vi "acoustic moderm processing.vi"(8 "error in (no error)":errorcluster, 9 "WRITE BUTTON":bool, 11 "Cluster":T1) -> (0 "error in (no error) 2":errorcluster, 1 "Modem Ready Status":bool, 2 "Data Tx/Rx":string, 3 "Data out":string)   [LabVIEW 2021]
panel:
  out "concatenated string":string
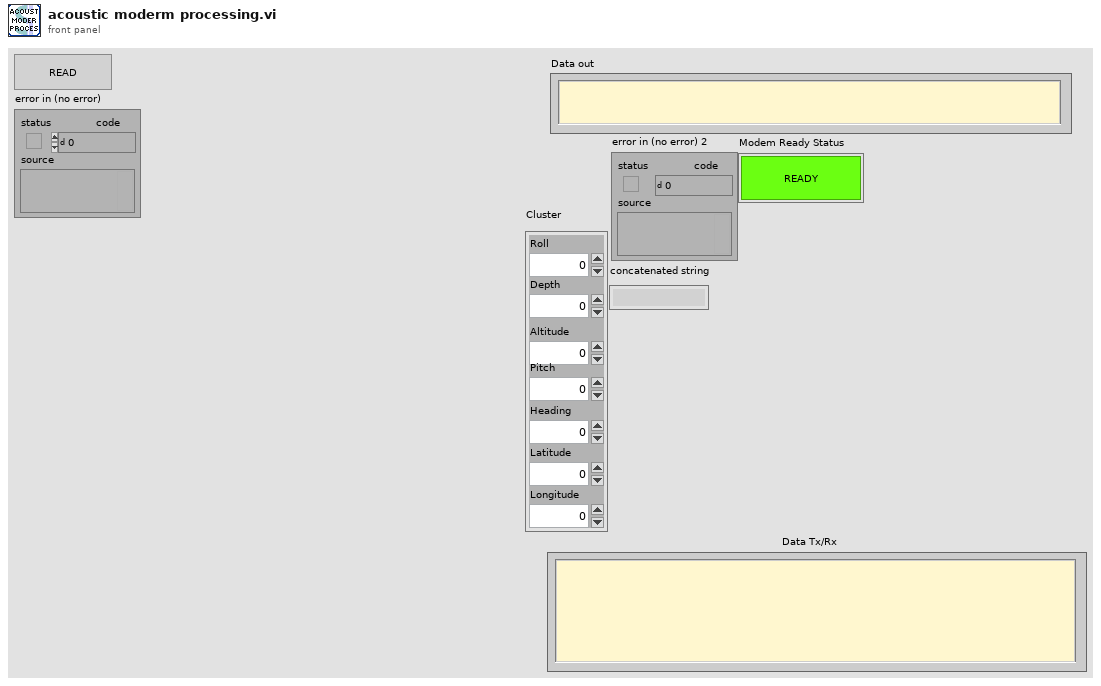
[diagram p1: front panel]
types:
  T1 = cluster{"Roll":sgl, "Depth":sgl, "Altitude":sgl, "Pitch":sgl, "Heading":sgl, "Latitude":sgl, "Longitude":sgl}
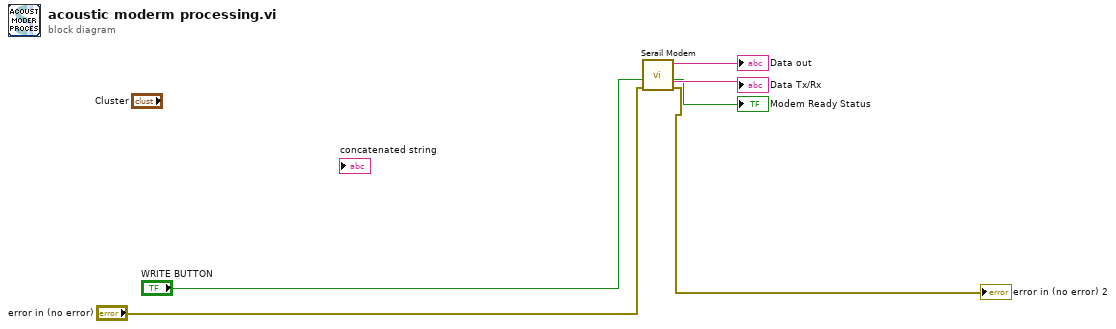
[diagram p0: block diagram]
diagram:
  n1 = call "Serail Modem.vi"("error in (no error)"="error in (no error)", "WRITE BUTTON"="WRITE BUTTON") -> ("error in (no error) 2"=→"error in (no error) 2":errorcluster, "Modem Ready Status"=→"Modem Ready Status":bool, "Data Tx/Rx"=→"Data Tx/Rx":string, "Data out"=→"Data out":string)  [unwired: 6 in]
